vi "HTML Report Get Case Matching.vi"(1 "string matching":T1=enum."system") -> (0 "match case":bool)   [LabVIEW 2017, in "NI_ReportGenerationCore.lvlib"]
uses:
  <vilib>/Utility/NIReport.llb/NI_ReportGenerationCore.lvlib
  <vilib>/Utility/NIReport.llb/HTML Report Case Matching.ctl
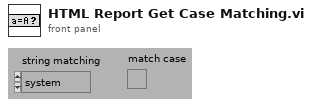
[diagram p1: front panel]
types:
  T1 = typedef "NI_ReportGenerationCore.lvlib/HTML Report Case Matching.ctl" = enum16{"a != A", "a == A", "system"}
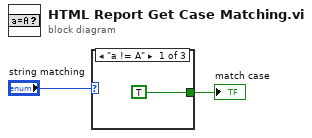
[diagram p0: block diagram]
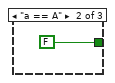
[diagram p2: hidden frame]
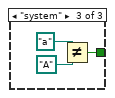
[diagram p3: hidden frame]
diagram:
  n1 = case shown="\"a != A\"" "string matching" {
    tunnel: [TRUE FALSE w5] -> w1
    frame "a != A" {
    }
    frame "a == A" {
    }
    frame "system" {
      n2 = Not Equal?(x=path "a", y=path "A") -> (x != y?=w5:bool)
    }
  }
  "match case" <- w1
